vi "GF_delayConfigSignal.vi"(1 "error in":errorcluster, 2 "Desired State":bool=TRUE, 3 "milliseconds to wait":u32, 4 "DAQmx Global Channel":refnum<k21>="DiagProbePSSwitch_P1-0") -> (0 "error out":errorcluster)   [LabVIEW 2009]
uses:
  <vilib>/DAQmx/write.llb/DAQmx Write (Digital Bool 1Line 1Point).vi
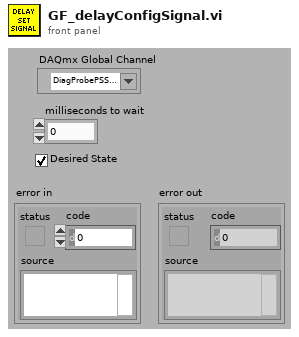
[diagram p1: front panel]
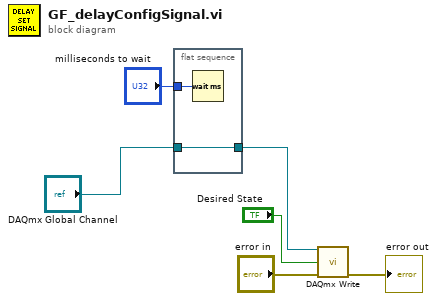
[diagram p0: block diagram]
diagram:
  n1 = flat-sequence {
    tunnel: "DAQmx Global Channel" -> [w8]
    tunnel: [w8] -> w3
    tunnel: "milliseconds to wait" -> [w7]
    frame #0 {
      n2 = Wait (ms)(milliseconds to wait=w7) -> ()  [unwired: 1 out]
    }
  }
  n3 = call-poly <vilib>:"DAQmx Write.vi"("task/channels in"=w3, "data"="Desired State", "error in"="error in") -> ("error out"=→"error out":errorcluster)  [unwired: 10 in, 2 out]
